vi "Parse Formula Node.vi"(2 "error in (no error)":errorcluster, 3 "formula":string, 4 "Variables Output":string[](array[string]), 5 "Variables Input":string[](array[string])) -> (0 "error out":errorcluster, 1 "Parsed Formula Node":T1 {"Y Values" format="%.2f"})   [LabVIEW 2020, in "NI_Gmath.lvlib"]
doc: "Analyzes Eval Formula Node VI inputs and yields an intermediate state as an input for the Eval Parsed Formula Node VI."
uses:
  NI_Gmath.lvlib
panel:
  # "Example:\n\n Variables Input: a and b\n Variables Output: x and y \n formula: x=a+b;y=a*b;"
  # "operator"
  # "register1"
  # "register2"
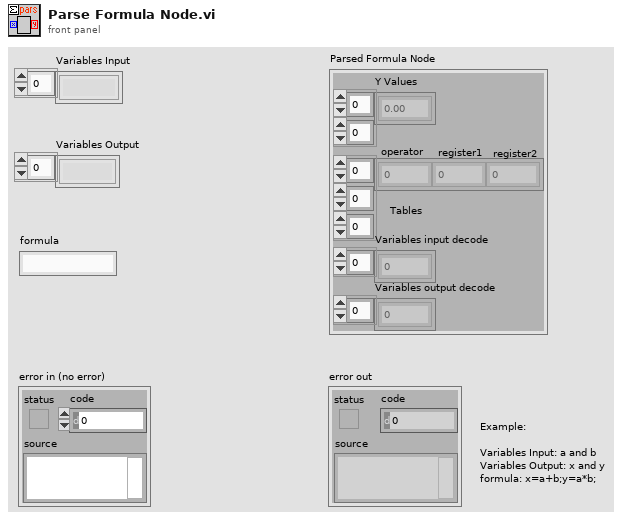
[diagram p1: front panel]
types:
  T1 = cluster{"Y Values":dbl[][], "Tables":i32[][][], "Variables input decode":i32[], "Variables output decode":i32[]}
  T2 = cluster{"Y Values":dbl[][], "Table":i32[][][], i32[], i32[]}
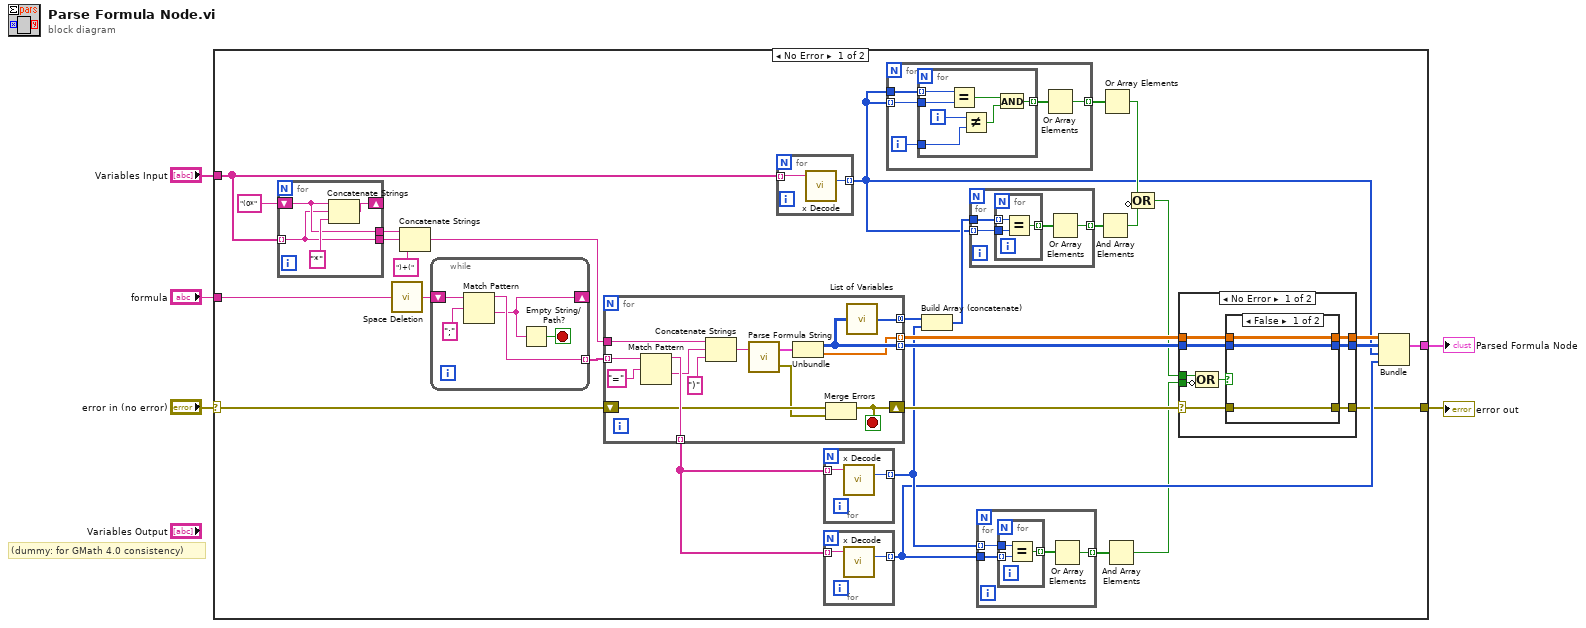
[diagram p0: block diagram]
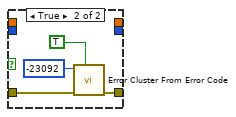
[diagram p2: hidden frame]
diagram:
  # "(dummy: for GMath 4.0 consistency)"
  n1 = case shown="No Error" "error in (no error)" {
    selector: "error in (no error)" -> [w12 w108]
    tunnel: "Variables Input" -> [w20 _]
    tunnel: "formula" -> [w16 _]
    tunnel: [w11 w108] -> w2
    tunnel: [w10 _] -> w1
    frame No Error {
      n2 = for {
        shift-right: [w43] -> _
        shift-left: "(0*" -> [w42]
        tunnel: w20 -> [w41] mode=indexing
        tunnel: [w42] -> w19
        tunnel: [w41] -> w18
        n3 = Concatenate Strings(w42, w41, "*") -> (w43:string)
      }
      n4 = call "Space Deletion.vi"("string with spaces"=w16) -> ("string without spaces"=w35:string)
      n5 = Concatenate Strings(w19, w18, ")+(") -> (w15:string)
      n6 = while {
        shift-left: w35 -> [w40]
        shift-right: [w37] -> _
        tunnel: [w38] -> w9 mode=indexing
        stop <- w39 stop-if-true
        n7 = Match Pattern(string=w40, regular expression=";") -> (before substring=w38:string, after substring=w37:string)  [unwired: 1 in, 2 out]
        n8 = Empty String/Path?(string/path=w37) -> (empty?=w39:bool)
      }
      n9 = for {
        tunnel: w9 -> [w107] mode=indexing
        tunnel: [w104] -> w33 mode=indexing
        tunnel: [w103] -> w34 mode=indexing
        tunnel: [w106] -> w14 mode=indexing
        shift-right: [w94] -> w32
        shift-left: w12 -> [w96]
        tunnel: w15 -> [w101]
        tunnel: [w98] -> w8 mode=concatenating
        stop <- w94 stop-if-true
        n10 = Match Pattern(string=w107, regular expression="=") -> (before substring=w106:string, after substring=w100:string)  [unwired: 1 in, 2 out]
        n11 = Concatenate Strings(w101, w100, ")") -> (w99:string)
        n12 = call "Parse Formula String.vi"("formula"=w99) -> ("error out"=w95:errorcluster, "Parsed Formula"=w105:cluster{"Table":i32[][], "Y Values":dbl[]})  [unwired: 1 in]
        n13 = Unbundle(w105) -> ("Table"=w104:i32[][], "Y Values"=w103:dbl[])
        n14 = Merge Errors(w96, w95) -> (w94:errorcluster)
        n15 = call "List of Variables.vi"("Table"=w104) -> ("List of variables"=w98:i32[])
      }
      n16 = for {
        tunnel: w20 -> [w46] mode=indexing
        tunnel: [w45] -> w22 mode=indexing
        n17 = call "x Decode.vi"("x string"=w46) -> ("number"=w45:i32)  [unwired: 1 in, 1 out]
      }
      n18 = for {
        tunnel: w14 -> [w93] mode=indexing
        tunnel: [w92] -> w25 mode=indexing
        n19 = call "x Decode.vi"("x string"=w93) -> ("number"=w92:i32)  [unwired: 1 in, 1 out]
      }
      n20 = for {
        tunnel: w14 -> [w91] mode=indexing
        tunnel: [w90] -> w13 mode=indexing
        n21 = call "x Decode.vi"("x string"=w91) -> ("number"=w90:i32)  [unwired: 1 in, 1 out]
      }
      n22 = for {
        tunnel: w22 -> [w51] mode=indexing
        tunnel: w22 -> [w50]
        tunnel: [w48] -> w28 mode=indexing
        i -> [w47]
        n23 = for {
          tunnel: w51 -> [w58]
          tunnel: w50 -> [w57] mode=indexing
          tunnel: [w52] -> w49 mode=indexing
          tunnel: w47 -> [w55]
          i -> [w56]
          n24 = Equal?(x=w57, y=w58) -> (x = y?=w53:bool)
          n25 = Not Equal?(x=w56, y=w55) -> (x != y?=w54:bool)
          n26 = And(x=w53, y=w54) -> (x .and. y?=w52:bool)
        }
        n27 = Or Array Elements(Boolean array=w49) -> (logical OR=w48:bool)
      }
      n28 = Build Array (concatenate)(w8, w25) -> (w29:i32[])
      n29 = for {
        tunnel: w22 -> [w62] mode=indexing
        tunnel: w29 -> [w61]
        tunnel: [w59] -> w30 mode=indexing
        n30 = for {
          tunnel: w62 -> [w65]
          tunnel: w61 -> [w64] mode=indexing
          tunnel: [w63] -> w60 mode=indexing
          n31 = Equal?(x=w64, y=w65) -> (x = y?=w63:bool)
        }
        n32 = Or Array Elements(Boolean array=w60) -> (logical OR=w59:bool)
      }
      n33 = for {
        tunnel: w13 -> [w86]
        tunnel: w25 -> [w85] mode=indexing
        tunnel: [w83] -> w31 mode=indexing
        n34 = for {
          tunnel: w86 -> [w89] mode=indexing
          tunnel: w85 -> [w88]
          tunnel: [w87] -> w84 mode=indexing
          n35 = Equal?(x=w88, y=w89) -> (x = y?=w87:bool)
        }
        n36 = Or Array Elements(Boolean array=w84) -> (logical OR=w83:bool)
      }
      n37 = And Array Elements(Boolean array=w30) -> (logical AND=w7:bool)
      n38 = Or Array Elements(Boolean array=w28) -> (logical OR=w26:bool)
      n39 = And Array Elements(Boolean array=w31) -> (logical AND=w6:bool)
      n40 = Compound Arithmetic op=OR(w26, invert w7) -> (w27:bool)
      n41 = case shown="No Error" w32 {
        selector: w32 -> [w70 w82]
        tunnel: [w74 _] -> w24
        tunnel: [w73 _] -> w23
        tunnel: w6 -> [w66 _]
        tunnel: w34 -> [w72 _]
        tunnel: w33 -> [w71 _]
        tunnel: [w69 w82] -> w11
        tunnel: w27 -> [w67 _]
        frame No Error {
          n42 = Compound Arithmetic op=OR(w67, invert w66) -> (w68:bool)
          n43 = case shown="False" w68 {
            tunnel: [w77 _] -> w74
            tunnel: [w76 _] -> w73
            tunnel: w72 -> [w77 _]
            tunnel: w71 -> [w76 _]
            tunnel: w70 -> [w75 w80]
            tunnel: [w75 w81] -> w69
            frame False {
            }
            frame True {
              n44 = call "Error Cluster From Error Code.vi"("show call chain? (False)"=TRUE, "error in (no error)"=w80, "error code (0)"=-23092) -> ("error out"=w81:errorcluster)  [unwired: 6 in]
            }
          }
        }
        frame Error {
        }
      }
      n45 = Bundle("Y Values"=w24, "Table"=w23, w22, w13) -> (w10:T2)  [unwired: 1 in]
    }
    frame Error {
    }
  }
  "error out" <- w2
  "Parsed Formula Node" <- w1
